vi "Calc-Exchanges.vi"(10 "Exchanges":T1[](array[typedef])) -> (0 "Lignes":refnum<class "Stock.lvclass">[](array[class]), 1 "Qtés restante par ligne":dbl[](array[numeric]), 2 "Total":dbl)   [LabVIEW 2012]
uses:
  Exchange/Exchange Parameters.ctl
  Exchange/Exchange Type Enum.ctl
  controls/Currencies.ctl
  Stock/Stock.lvclass
  Stock/Stock Parameters.ctl
  Stock/Stock.lvclass/Stock.ctl
  Exchange/Exchange.lvclass
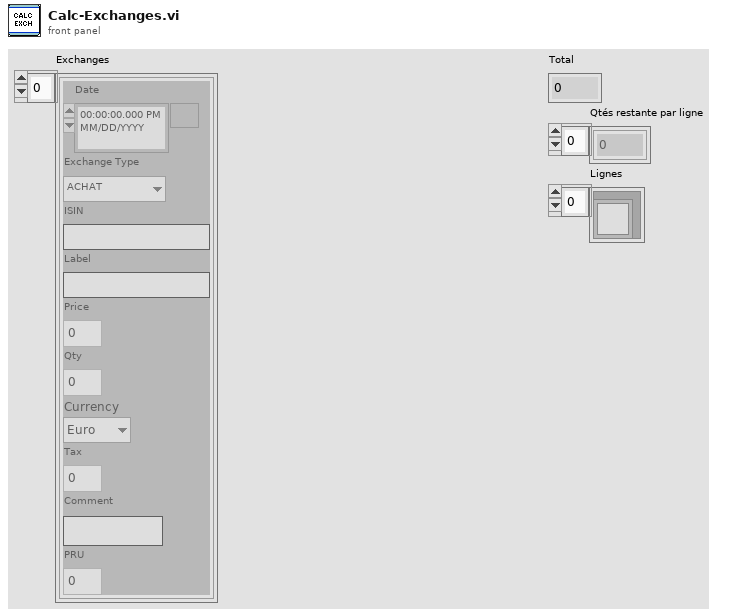
[diagram p1: front panel]
types:
  T1 = typedef "Exchange Parameters.ctl" = cluster{"Date":timestamp, "Exchange Type":T2, "ISIN":string, "Label":string, "Price":dbl, "Qty":dbl, "Currency":T3, "Tax":dbl, "Comment":string, "PRU":dbl}
  T2 = typedef "Exchange.lvclass/Exchange Type Enum.ctl" = enum16{"ACHAT", "VENTE"}
  T3 = typedef "Currencies.ctl" = enum16{"Euro", "Dollar", "Yen", "RIM", "CHF"}
  T4 = typedef "Stock.lvclass/Stock Parameters.ctl" = cluster{"Label":string, "Symbol":string, "Dividend":dbl, "Currency":T3, "ISIN":string, "Symbol_Suffix":string, "Last Price":dbl, "Dividend-Date":string, "Change (%)":dbl}
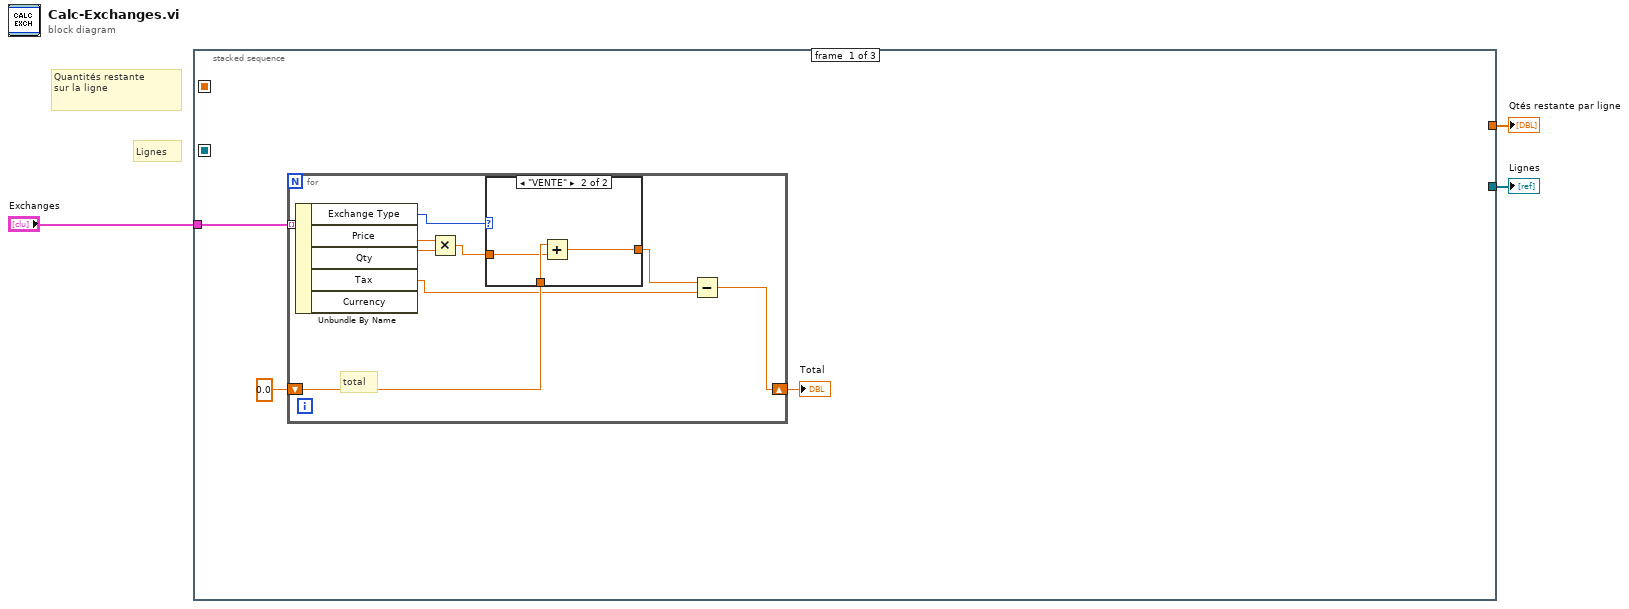
[diagram p0: block diagram]
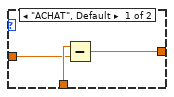
[diagram p2: hidden frame]
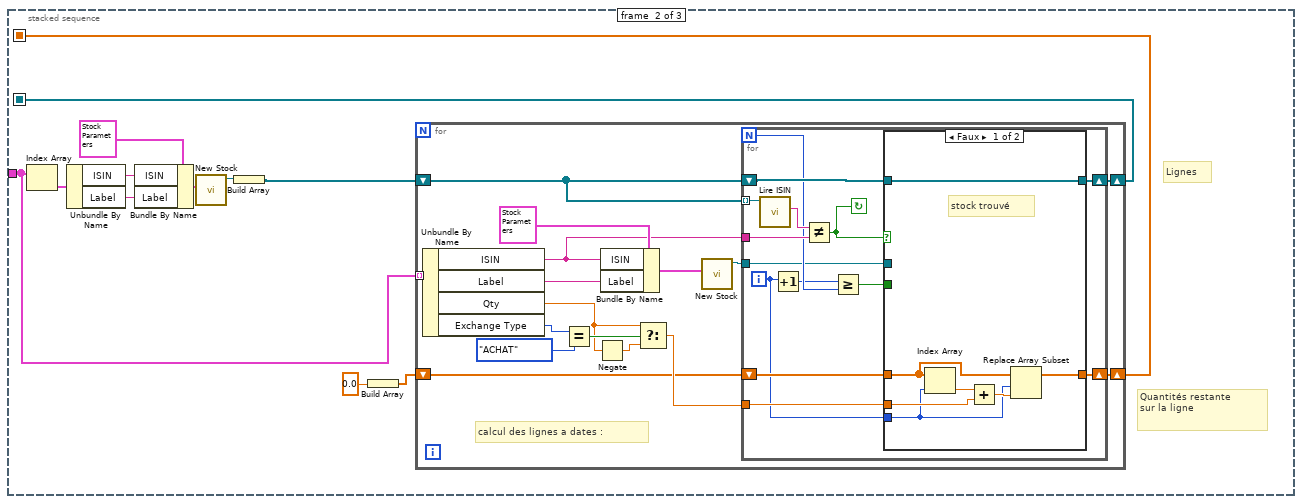
[diagram p3: hidden frame]
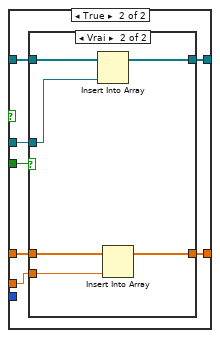
[diagram p4: hidden frame]
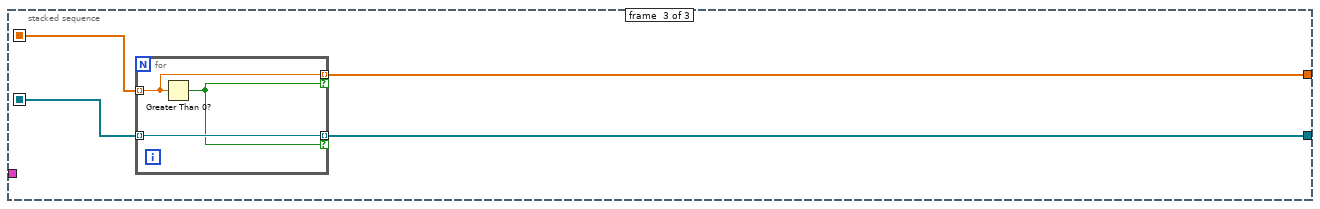
[diagram p6: hidden frame]
diagram:
  # "Quantités restante \nsur la ligne"
  # "Lignes"
  n1 = stacked-sequence {
    seq-local: [_ w23 _] -> [_ _ w89]
    seq-local: [_ w22 _] -> [_ _ w88]
    tunnel: "Exchanges" -> [w5 w25 _]
    tunnel: [_ _ w87] -> w2
    tunnel: [_ _ w86] -> w1
    frame #0 {
      n2 = for {
        tunnel: w5 -> [w15] mode=indexing
        shift-right: [w8] -> w4
        shift-left: 0.0 -> [w13]
        # "total"
        n3 = Unbundle By Name(w15) -> ("Exchange Type"=w14:T2, "Price"=w12:dbl, "Qty"=w11:dbl, "Tax"=w7:dbl)  [unwired: 1 out]
        n4 = Multiply(x=w12, y=w11) -> (x*y=w10:dbl)
        n5 = case shown="\"VENTE\"" w14 {
          tunnel: w13 -> [w18 w21]
          tunnel: w10 -> [w16 w19]
          tunnel: [w17 w20] -> w9
          frame "ACHAT", Default {
            n6 = Subtract(x=w18, y=w16) -> (x-y=w17:dbl)
          }
          frame "VENTE" {
            n7 = Add(x=w21, y=w19) -> (x+y=w20:dbl)
          }
        }
        n8 = Subtract(x=w9, y=w7) -> (x-y=w8:dbl)
      }
      "Total" <- w4
    }
    frame #1 {
      # "Lignes"
      # "Quantités restante \nsur la ligne"
      n9 = Index Array(array=w25) -> (element=w33:T1)  [unwired: 1 in]
      n10 = Unbundle By Name(w33) -> ("ISIN"=w31:string, "Label"=w30:string)
      n11 = Bundle By Name(cluster=T4 {"Label"="", "Symbol"="SU", "Dividend"=0.0, "Currency"=enum."Euro", "ISIN"="", "Symbol_Suffix"=".PA", "Last Price"=0.0, "Dividend-Date"="", "Change (%)"=0.0} ("Parameters"), "ISIN"=w31, "Label"=w30) -> (w29:T4)
      n12 = call "New Stock.vi"("Parameters"=w29) -> ("Stock en sortie"=w28:refnum<class "Stock.lvclass">)  [unwired: 9 in, 1 out]
      n13 = Build Array(w28) -> (w24:refnum<class "Stock.lvclass">[])
      n14 = Build Array(0.0) -> (w27:dbl[])
      n15 = for {
        tunnel: w25 -> [w49] mode=indexing
        shift-right: [w42] -> w22
        shift-left: w24 -> [w48]
        shift-right: [w35] -> w23
        shift-left: w27 -> [w34]
        # "calcul des lignes a dates :"
        n16 = Unbundle By Name(w49) -> ("ISIN"=w46:string, "Label"=w43:string, "Qty"=w38:dbl, "Exchange Type"=w41:T2)
        n17 = Equal?(x=w41, y=Exchange_Type_Enum."ACHAT") -> (x = y?=w39:bool)
        n18 = Negate(x=w38) -> (-x=w37:dbl)
        n19 = Bundle By Name(cluster=T4 {"Label"="", "Symbol"="SU", "Dividend"=0.0, "Currency"=enum."Euro", "ISIN"="", "Symbol_Suffix"=".PA", "Last Price"=0.0, "Dividend-Date"="", "Change (%)"=0.0} ("Parameters"), "ISIN"=w46, "Label"=w43) -> (w45:T4)
        n20 = Select(t=w38, s=w39, f=w37) -> (s? t:f=w36:dbl)
        n21 = call "New Stock.vi"("Parameters"=w45) -> ("Stock en sortie"=w44:refnum<class "Stock.lvclass">)  [unwired: 9 in, 1 out]
        n22 = for {
          N -> [w59]
          tunnel: w48 -> [w63] mode=indexing
          tunnel: w46 -> [w61]
          tunnel: w44 -> [w51]
          shift-right: [w58] -> w42
          shift-left: w48 -> [w60]
          tunnel: w36 -> [w55]
          shift-right: [w56] -> w35
          shift-left: w34 -> [w57]
          i -> [w54]
          stop <- w52 continue-if-true
          n23 = call "Lire ISIN.vi"("Share en entrée"=w63) -> ("ISIN"=w62:string)  [unwired: 8 in, 2 out]
          n24 = Increment(x=w54) -> (x+1=w53:i32)
          n25 = Not Equal?(x=w62, y=w61) -> (x != y?=w52:bool)
          n26 = Greater Or Equal?(x=w53, y=w59) -> (x >= y?=w50:bool)
          n27 = case shown="Faux" w52 {
            tunnel: w60 -> [w70 w76]
            tunnel: w57 -> [w65 w75]
            tunnel: [w70 w74] -> w58
            tunnel: [w64 w73] -> w56
            tunnel: w55 -> [w69 w71]
            tunnel: w54 -> [w66 _]
            tunnel: w51 -> [_ w72]
            tunnel: w50 -> [_ w77]
            frame False {
              # "stock trouvé"
              n28 = Index Array(array=w65, index=w66) -> (element=w68:dbl)
              n29 = Add(x=w68, y=w69) -> (x+y=w67:dbl)
              n30 = Replace Array Subset(array=w65, new element=w67, index=w66) -> (w64:dbl[])
            }
            frame True {
              n31 = case shown="Vrai" w77 {
                tunnel: w76 -> [w79 w85]
                tunnel: w75 -> [w78 w82]
                tunnel: [w79 w84] -> w74
                tunnel: [w78 w81] -> w73
                tunnel: w72 -> [_ w83]
                tunnel: w71 -> [_ w80]
                frame False {
                }
                frame True {
                  n32 = Insert Into Array(array=w85, new element=w83) -> (w84:refnum<class "Stock.lvclass">[])  [unwired: 1 in]
                  n33 = Insert Into Array(array=w82, new element=w80) -> (w81:dbl[])  [unwired: 1 in]
                }
              }
            }
          }
        }
      }
    }
    frame #2 {
      n34 = for {
        tunnel: w88 -> [w92] mode=indexing
        tunnel: w89 -> [w91] mode=indexing
        tunnel: [w92] -> w86 mode=indexing if=w90
        tunnel: [w91] -> w87 mode=indexing if=w90
        n35 = Greater Than 0?(x=w91) -> (x > 0?=w90:bool)
      }
    }
  }
  "Qtés restante par ligne" <- w2
  "Lignes" <- w1
